vi "DCT.vi"   [LabVIEW 2018, in "NI_AALPro.lvlib"]
doc: "Computes the Discrete Cosine Transform (DCT) of the input sequence <B>X</B>. Wire data to the <B>X</B> input to determine the polymorphic instance to use or manually select the instance."
uses:
  <vilib>/Analysis/NI_AALPro.lvlib
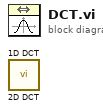
[diagram p0: block diagram]
diagram:
  n1 = call "2D DCT.vi"() -> ()  [unwired: 10 in, 2 out]
  n2 = call "1D DCT.vi"() -> ()  [unwired: 10 in, 2 out]
